vi "IL Sample Push State.vi"(4 "Add to (Deny)":T2, 5 "Ignore (F)":bool, 7 "Stop Self on IL? (T)":bool=TRUE, 8 "error in (no error)":errorcluster, 9 "States":T1[](array[typedef]), 10 "Pass/Seize":enum16{"Pass", "Seize"}(ring), 11 "Interlock Chain in":refnum<class "Interlock Chain.lvclass">) -> (0 "error out":errorcluster, 2 "IL Sample Push State":refnum<class "Interlock.lvclass">, 3 "Interlock Chain out":refnum<class "Interlock Chain.lvclass">)   [LabVIEW 2015, in "cRIO-Carbondioxide.lvlib" / "cRIO-CO2.lvlib" / "cRIO-CO2.lvclass"]
uses:
  cRIO-CO2.lvclass
  Interlocks/Interlock Chain/Interlock Chain.lvclass
  Interlocks/Controls/Add IL to -Enumerator.ctl
  Interlocks/Interlock/Interlock.lvclass
  Controls/Sample Push State Enumerator.ctl
  Interlocks/Interlock U16/Seize/IL U16 Seize.lvclass
  Interlocks/Interlock U16/Seize/IL U16 Seize.lvclass/IL U16 Seize.ctl
  Interlocks/Interlock U16/Pass/IL U16 Pass.lvclass
  Interlocks/Interlock U16/Pass/IL U16 Pass.lvclass/IL U16 Pass.ctl
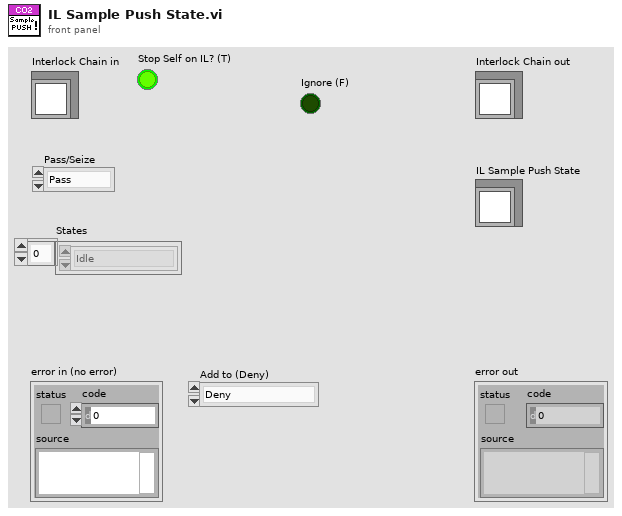
[diagram p1: front panel]
types:
  T1 = typedef "Sample Push State Enumerator.ctl" = enum16{"Undefined", "Initialize", "Dilute", "Close Transfer Line", "Start Heaters", "Warm Up Syringe", "Ready to Push", "Push", "Initiate Stash", "Stash", "Complete", "Abort", "Idle", "Error"}
  T2 = typedef "Add IL to -Enumerator.ctl" = enum16{"Deny", "Allow", "None"}
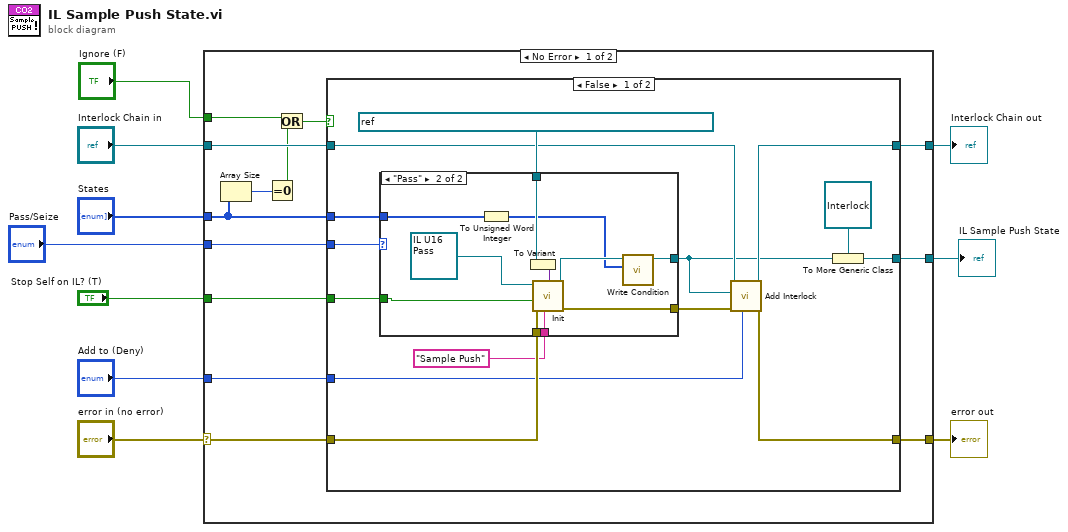
[diagram p0: block diagram]
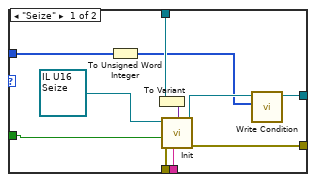
[diagram p2: hidden frame]
diagram:
  n1 = case shown="No Error" "error in (no error)" {
    selector: "error in (no error)" -> [w21 w63]
    tunnel: [w20 w63] -> w9
    tunnel: [w22 w62] -> w7
    tunnel: "Interlock Chain in" -> [w23 w62]
    tunnel: "Add to (Deny)" -> [w19 _]
    tunnel: [w18 _] -> w5
    tunnel: "Stop Self on IL? (T)" -> [w17 _]
    tunnel: "Ignore (F)" -> [w16 _]
    tunnel: "States" -> [w15 _]
    tunnel: "Pass/Seize" -> [w11 _]
    frame No Error {
      n2 = Array Size(array=w15) -> (size(s)=w13:i32)
      n3 = Equal To 0?(x=w13) -> (x = 0?=w12:bool)
      n4 = Or(x=w16, y=w12) -> (x .or. y?=w14:bool)
      n5 = case shown="False" w14 {
        tunnel: w23 -> [w36 w61]
        tunnel: [w35 w61] -> w22
        tunnel: w21 -> [w34 w60]
        tunnel: [w33 w60] -> w20
        tunnel: w19 -> [w32 _]
        tunnel: [w30 _] -> w18
        tunnel: w17 -> [w28 _]
        tunnel: w15 -> [w26 _]
        tunnel: w11 -> [w25 _]
        frame False {
          n6 = case shown="\"Pass\"" w25 {
            tunnel: refnum<k21> "ni.var.psp://10.2.0.20/AMS Gas SHV/Sample Push/State" ("SHV") -> [w47 w58]
            tunnel: w34 -> [w46 w57]
            tunnel: [w45 w56] -> w31
            tunnel: w28 -> [w38 w49]
            tunnel: [w43 w54] -> w27
            tunnel: w26 -> [w41 w52]
            tunnel: "Sample Push" ("Name (SHV Name if empty)") -> [w39 w50]
            frame "Seize" {
              n7 = To Unsigned Word Integer(number=w41) -> (unsigned 16bit integer=w40:u16[])
              n8 = To Variant(anything=w47) -> (Variant=w44:variant)
              n9 = call-dynamic "Init.vi"("Name (SHV Name if empty)"=w39, "SHV"=w44, "error in (no error)"=w46, "Stop Self on IL? (T)"=w38, "Interlock in"=refnum<class "IL U16 Seize.lvclass"> refnum ("Interlock Range.lvclass")) -> ("error out"=w43:errorcluster, "Interlock out"=w42:refnum<class "IL U16 Seize.lvclass">)  [unwired: 5 in]
              n10 = call "Write Condition.vi"("Deny"=w40, "IL U16 Deny in"=w42) -> ("IL U16 Deny out"=w45:refnum<class "IL U16 Seize.lvclass">)  [unwired: 9 in]
            }
            frame "Pass" {
              n11 = To Unsigned Word Integer(number=w52) -> (unsigned 16bit integer=w51:u16[])
              n12 = To Variant(anything=w58) -> (Variant=w55:variant)
              n13 = call-dynamic "Init.vi"("Name (SHV Name if empty)"=w50, "SHV"=w55, "error in (no error)"=w57, "Stop Self on IL? (T)"=w49, "Interlock in"=refnum<class "IL U16 Pass.lvclass"> refnum ("Interlock Range.lvclass")) -> ("error out"=w54:errorcluster, "Interlock out"=w53:refnum<class "IL U16 Pass.lvclass">)  [unwired: 5 in]
              n14 = call "Write Condition.vi"("Allow"=w51, "IL U16 Allow in"=w53) -> ("IL U16 Allow out"=w56:refnum<class "IL U16 Pass.lvclass">)  [unwired: 9 in]
            }
          }
          n15 = call "Add Interlock.vi"("Add to (Deny)"=w32, "error in (no error)"=w27, "Interlock.lvclass"=w31, "Interlock Chain in"=w36) -> ("error out"=w33:errorcluster, "Interlock Chain out"=w35:refnum<class "Interlock Chain.lvclass">)  [unwired: 6 in]
          n16 = To More Generic Class(target class=refnum<class "Interlock.lvclass"> refnum ("Interlock.lvclass"), reference=w31) -> (generic class reference=w30:refnum<class "Interlock.lvclass">)
        }
        frame True {
        }
      }
    }
    frame Error {
    }
  }
  "error out" <- w9
  "Interlock Chain out" <- w7
  "IL Sample Push State" <- w5
